vi "TEST Object Manual Bounds.vi"() -> ()   [LabVIEW 2021, in "IObject.lvclass"]
uses:
  IObject.lvclass
  <vilib>/Utility/miscctls.llb/LVRectTypeDef.ctl
  Object/Object.lvclass
panel:
  in  "Bounds":T1={"Left"=100, "Top"=50, "Right"=200, "Bottom"=150}
  in  "OK Button":bool
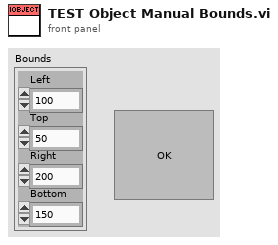
[diagram p1: front panel]
types:
  T1 = typedef "LVRectTypeDef.ctl" = cluster{"Left":i16, "Top":i16, "Right":i16, "Bottom":i16}
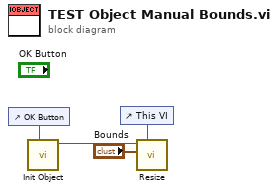
[diagram p0: block diagram]
diagram:
  n1 = control-ref of="OK Button"() -> (w4:refnum<vi>)
  n2 = call "Init Object.vi"("GObj Refnum"=w4) -> ("MMI Scaling out"=w3:refnum<class "Object.lvclass">)  [unwired: 9 in, 1 out]
  n3 = control-ref of="This VI"() -> (w2:refnum<vi>)
  n4 = call-dynamic "Resize.vi"("VI Refnum"=w2, "Bounds"="Bounds", "MMI Scaling in"=w3) -> ()  [unwired: 6 in, 3 out]
